vi "Compumet.vi"() -> ()   [LabVIEW 2010]
uses:
  file/file command.ctl
  serial commands.ctl
  toolbar icons/log data.ctl
  toolbar icons/file comment.ctl
  Spectrophotometer/settings.ctl
panel:
  in  "Serial Configure":T1={"integration time"=10000.0, "rinse time"=9600.0, "sample time"=8.0, "sample type"=0} {"sample type" items=["Sample Cuvet", "Sipper Cell", "No Dialog"]; "sample time" min=0.0 max=100.0 step=1.0 format="%.1f"; "rinse time" min=0.0 max=100.0 step=1.0 format="%.1f"; "integration time" format="%.1f"}
  out "Read line":string
  in  "Quit":bool
  in  "Monitor sample":bool
  in  "File Comment":T2
  in  "Log Data":T3
  in  "stop sampling":bool
  out "quit":bool=TRUE
  in  "Serial Port":refnum<visa-resource-name>
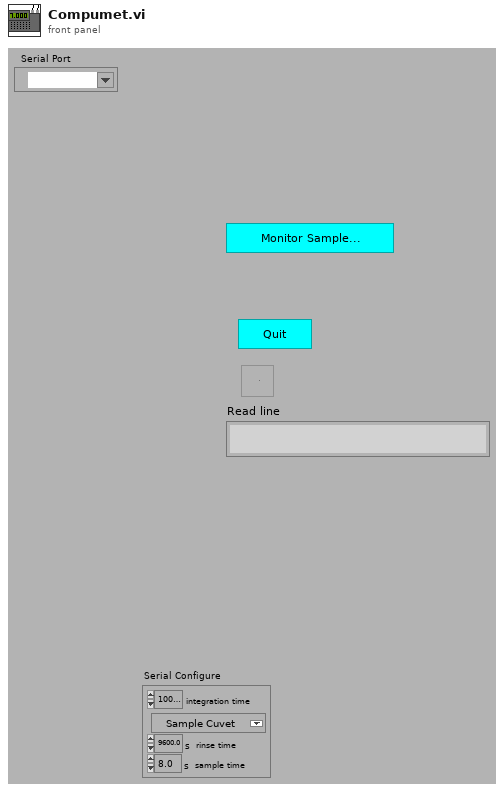
[diagram p1: front panel]
types:
  T1 = typedef "settings.ctl" = cluster{"integration time":sgl, "rinse time":dbl[unit], "sample time":dbl[unit], "sample type":u16}
  T2 = typedef "file comment.ctl" = bool
  T3 = typedef "log data.ctl" = bool
  T4 = typedef "serial commands.ctl" = enum16{"configure", "VISA resource", "write line", "read line", "Clear buffer", "close"}
  T5 = typedef "file command.ctl" = enum16{"Open Default", "Open", "Write  num ", "Write text", "Write comment", "Read num", "Read text", "Close"}
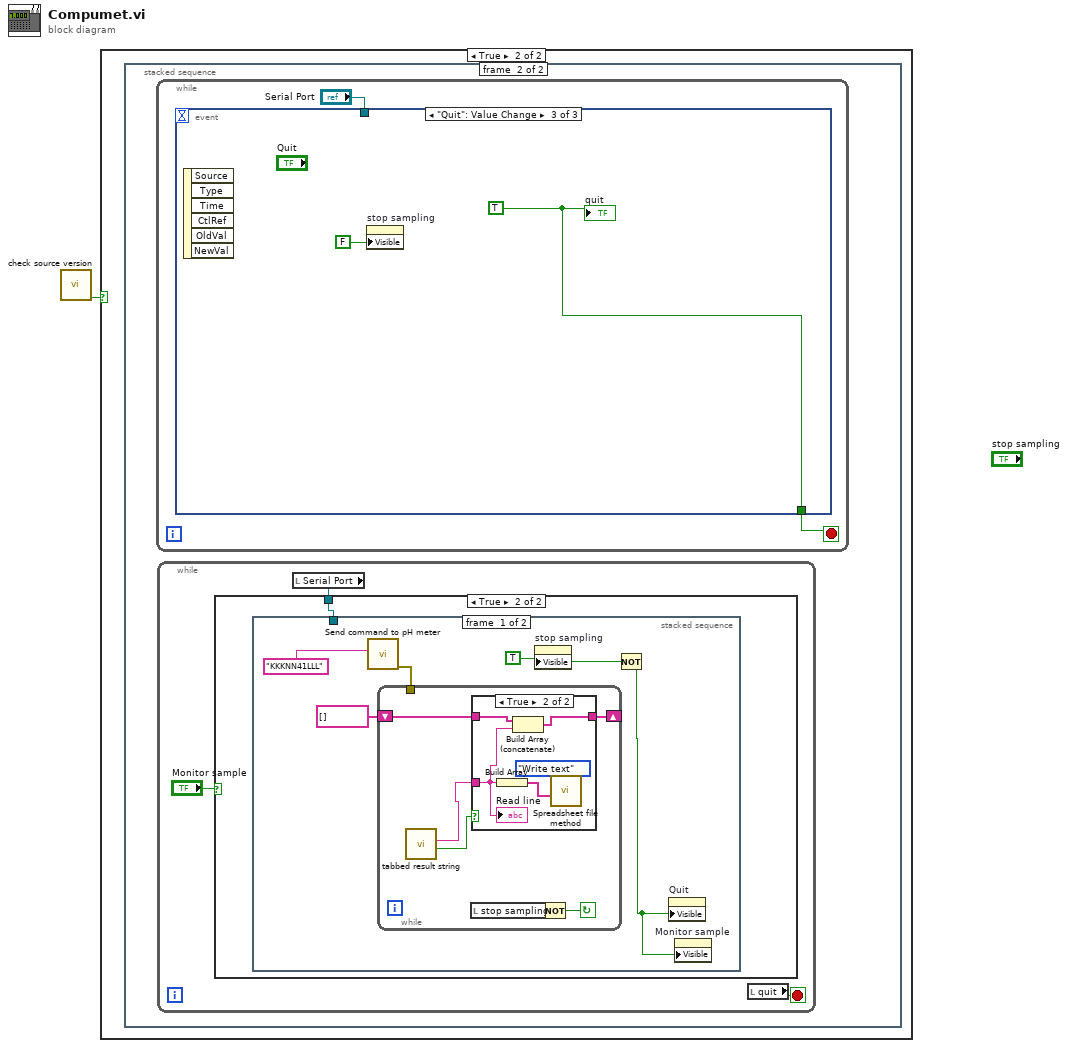
[diagram p0: block diagram]
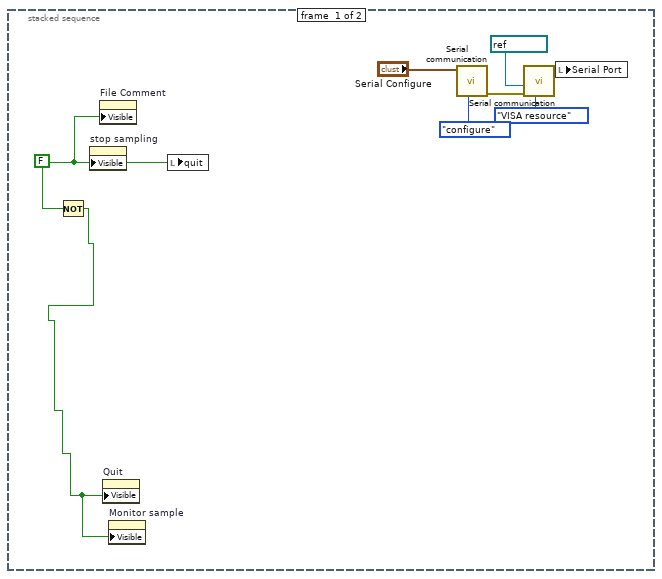
[diagram p3: hidden frame]
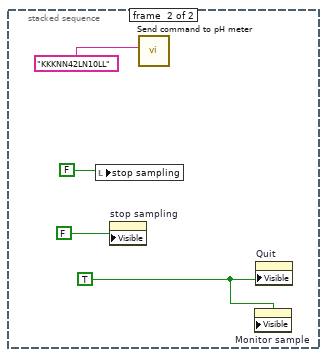
[diagram p6: hidden frame]
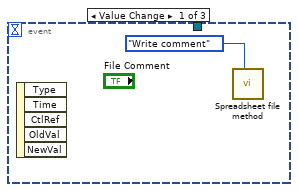
[diagram p7: hidden frame]
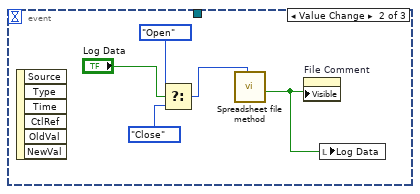
[diagram p8: hidden frame]
diagram:
  n1 = call "check source version.vi"() -> ("continue running?"=w1:bool)  [unwired: 2 in, 3 out]
  n2 = case shown="True" w1 {
    frame False {
    }
    frame True {
      n3 = stacked-sequence {
        frame #0 {
          w3 = FALSE
          n4 = Not(x=w3) -> (.not. x?=w2:bool)
          n5 = property on="stop sampling" class="Bool (strict)"("Visible"=w3) -> ()  [unwired: 2 in, 2 out]
          n6 = property on="File Comment" class="Bool"("Visible"=w3) -> ()  [unwired: 2 in, 2 out]
          n7 = property on="Quit" class="Bool"("Visible"=w2) -> ()  [unwired: 2 in, 2 out]
          n8 = property on="Monitor sample" class="Bool"("Visible"=w2) -> ()  [unwired: 2 in, 2 out]
          n9 = local write "quit"(w3) -> ()
          n10 = call <userlib>:"Serial communication.vi"("serial commands"=serial_commands."configure", "Serial Configure"="Serial Configure") -> ("error out"=w7:errorcluster)  [unwired: 3 in, 3 out]
          n11 = call <userlib>:"Serial communication.vi"("serial commands"=serial_commands."VISA resource", "error in (no error)"=w7, "Serial Port"=refnum<visa-resource-name> "COM1") -> ("Serial Port 2"=w5:refnum<visa-resource-name>)  [unwired: 2 in, 3 out]
          n12 = local write "Serial Port"(w5) -> ()
        }
        frame #1 {
          n13 = while {
            stop <- w35 stop-if-true
            n14 = event shown="[2] \"Quit\": Value Change" {
              selector: _ -> [_ _ _]
              dyn-events: _ -> [_ _ _]
              timeout: _ -> [_ _ _]
              tunnel: "Serial Port" -> [_ _ _]
              tunnel: [_ _ w43] -> w35
              event Value Change {
                n15 = event-data() -> ()  [unwired: 1 in, 5 out]
                n16 = call "Spreadsheet file method.vi"("File command"=file_command."Write comment") -> ()  [unwired: 6 in, 3 out]
              }
              event Value Change {
                n17 = event-data() -> ()  [unwired: 1 in, 6 out]
                n18 = Select(t=file_command."Open" ("File command"), s="Log Data", f=file_command."Close" ("File command")) -> (s? t:f=w42:T5)
                n19 = call "Spreadsheet file method.vi"("File command"=w42) -> ("Valid File"=w38:bool)  [unwired: 6 in, 2 out]
                n20 = property on="File Comment" class="Bool"("Visible"=w38) -> ()  [unwired: 2 in, 2 out]
                n21 = local write "Log Data"(w38) -> ()
              }
              event "Quit": Value Change {
                w43 = TRUE
                n22 = event-data() -> ()  [unwired: 1 in, 6 out]
                n23 = property on="stop sampling" class="Bool (strict)"("Visible"=FALSE) -> ()  [unwired: 2 in, 2 out]
                "quit" <- w43
              }
            }
          }
          n24 = while {
            stop <- w12 stop-if-true
            n25 = local read "Serial Port"() -> (w10:refnum<visa-resource-name>)
            n26 = case shown="True" "Monitor sample" {
              tunnel: w10 -> [_ w13]
              frame False {
              }
              frame True {
                n27 = stacked-sequence {
                  tunnel: w13 -> [_ _]
                  frame #0 {
                    w18 = TRUE
                    n28 = call "Send command to pH meter"("string to write"="KKKNN41LLL") -> ("error out"=w14:errorcluster)  [unwired: 9 in, 1 out]
                    n29 = while {
                      shift-right: [w21] -> _
                      shift-left: string[] [] -> [w22]
                      tunnel: w14 -> [_]
                      stop <- w24 continue-if-true
                      n30 = call "tabbed result string.vi"() -> ("read success"=w19:bool, "tabbed string"=w20:string)  [unwired: 10 in]
                      n31 = local read "stop sampling"() -> (w23:bool)
                      n32 = case shown="True" w19 {
                        tunnel: w20 -> [_ w27]
                        tunnel: w22 -> [w25 w28]
                        tunnel: [w25 w26] -> w21
                        frame False {
                        }
                        frame True {
                          n33 = Build Array(w27) -> (w29:string[])
                          n34 = Build Array (concatenate)(w28, w27) -> (w26:string[])
                          n35 = call "Spreadsheet file method.vi"("File command"=file_command."Write text", "1D string"=w29) -> ()  [unwired: 5 in, 3 out]
                          "Read line" <- w27
                        }
                      }
                      n36 = Not(x=w23) -> (.not. x?=w24:bool)
                    }
                    n37 = property on="stop sampling" class="Bool (strict)"("Visible"=w18) -> ()  [unwired: 2 in, 2 out]
                    n38 = Not(x=w18) -> (.not. x?=w17:bool)
                    n39 = property on="Quit" class="Bool"("Visible"=w17) -> ()  [unwired: 2 in, 2 out]
                    n40 = property on="Monitor sample" class="Bool"("Visible"=w17) -> ()  [unwired: 2 in, 2 out]
                  }
                  frame #1 {
                    w31 = TRUE
                    n41 = local write "stop sampling"(FALSE) -> ()
                    n42 = property on="stop sampling" class="Bool (strict)"("Visible"=FALSE) -> ()  [unwired: 2 in, 2 out]
                    n43 = call "Send command to pH meter"("string to write"="KKKNN42LN10LL") -> ()  [unwired: 9 in, 2 out]
                    n44 = property on="Monitor sample" class="Bool"("Visible"=w31) -> ()  [unwired: 2 in, 2 out]
                    n45 = property on="Quit" class="Bool"("Visible"=w31) -> ()  [unwired: 2 in, 2 out]
                  }
                }
              }
            }
            n46 = local read "quit"() -> (w12:bool)
          }
        }
      }
    }
  }
